vi "Labview查看CPU、内存使用情况.vi"() -> (3 "硬件负载":T1 {"硬盘负载" format="%#.1g%"; "内存负载" format="%#.1g%"; "CPU负荷" format="%#_6g%"; "CPU各核心负载" format="%.0f%"})   [LabVIEW 2017]
uses:
  <resource>/objmgr/nisysapi.rc
panel:
  out "System Inf":T2
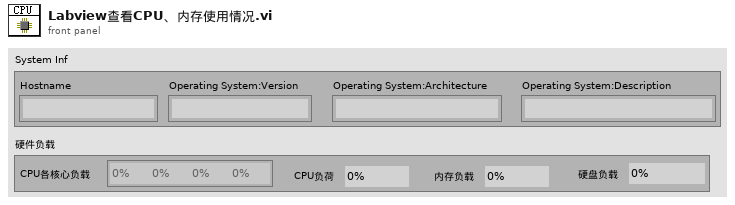
[diagram p1: front panel]
types:
  T1 = cluster{"CPU各核心负载":u32[], "CPU负荷":dbl, "内存负载":dbl, "硬盘负载":dbl}
  T2 = cluster{"Hostname":string, "Operating System:Version":string, "Operating System:Architecture":string, "Operating System:Description":string}
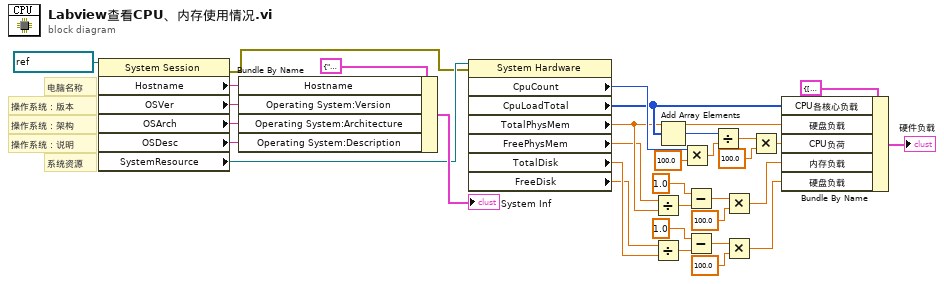
[diagram p0: block diagram]
diagram:
  # "系统资源"
  # "操作系统：说明"
  # "操作系统：架构"
  # "操作系统：版本"
  # "电脑名称"
  n1 = property class="System Session"(reference=refnum<k21> "localhost" ("Target (localhost)")) -> (error out=w2:errorcluster, "Hostname"=w6:string, "OSVer"=w7:string, "OSArch"=w8:string, "OSDesc"=w9:string, "SystemResource"=w3:refnum<k20>)  [unwired: 1 in, 1 out]
  n2 = Bundle By Name(cluster=T2 {"Hostname"="PC-201906191007", "Operating System:Version"="10.0.17763", "Operating System:Architecture"="Windows x64", "Operating System:Description"="Microsoft Windows 10 专业版"} ("System Inf"), "Hostname"=w6, "Operating System:Version"=w7, "Operating System:Architecture"=w8, "Operating System:Description"=w9) -> (→"System Inf":T2)
  n3 = property class="System Hardware"(reference=w3, error in=w2) -> ("CpuCount"=w20:i32, "CpuLoadTotal"=w19:u32[], "TotalPhysMem"=w18:dbl, "FreePhysMem"=w17:dbl, "TotalDisk"=w16:dbl, "FreeDisk"=w15:dbl)  [unwired: 2 out]
  n4 = Divide(x=w17, y=w18) -> (x/y=w28:dbl)
  n5 = Divide(x=w15, y=w16) -> (x/y=w21:dbl)
  n6 = Add Array Elements(numeric array=w19) -> (sum=w31:u32)
  n7 = Multiply(x=w20, y=100.0) -> (x*y=w32:dbl)
  n8 = Subtract(x=1.0, y=w28) -> (x-y=w25:dbl)
  n9 = Subtract(x=1.0, y=w21) -> (x-y=w24:dbl)
  n10 = Divide(x=w31, y=w32) -> (x/y=w30:dbl)
  n11 = Multiply(x=w25, y=100.0) -> (x*y=w12:dbl)
  n12 = Multiply(x=w24, y=100.0) -> (x*y=w11:dbl)
  n13 = Multiply(x=w30, y=100.0) -> (x*y=w13:dbl)
  n14 = Bundle By Name(cluster=T1 {"CPU各核心负载"=[9, 25, 21, 12], "CPU负荷"=16.75, "内存负载"=56.48655429645182, "硬盘负载"=40.29586920045074} ("硬件负载"), "CPU各核心负载"=w19, "硬盘负载"=w18, "CPU负荷"=w13, "内存负载"=w12, "硬盘负载"=w11) -> (→"硬件负载":T1)
